vi "Colour.vi"(9 "result":string, 11 "colourRef":refnum<vi>) -> (3 "colourRef 2":refnum<vi>)   [LabVIEW 2020]
panel:
  in  "黄灯":bool
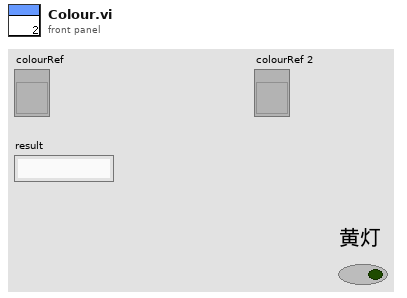
[diagram p1: front panel]
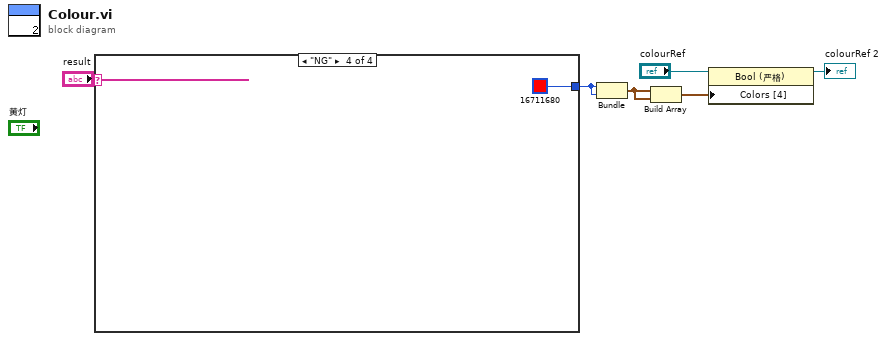
[diagram p0: block diagram]
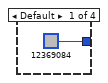
[diagram p2: hidden frame]
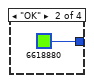
[diagram p3: hidden frame]
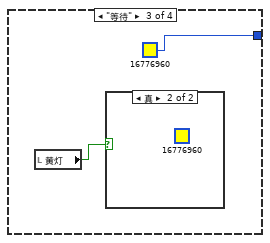
[diagram p4: hidden frame]
diagram:
  n1 = case shown="\"NG\"" "result" {
    tunnel: [u32 12369084 u32 6618880 u32 16776960 u32 16711680] -> w6
    frame Default {
    }
    frame "OK" {
    }
    frame "等待" {
      n2 = local read "黄灯"() -> (w10:bool)
      n3 = case shown="真" w10 {
        frame False {
        }
        frame True {
          (unwired) u32 16776960
        }
      }
    }
    frame "NG" {
    }
  }
  n4 = Bundle(w6, w6) -> (w5:cluster{u32, u32})  [unwired: 1 in]
  n5 = Build Array(w5, w5) -> (w1:cluster{u32, u32}[])
  n6 = property class="Bool (严格)"(reference="colourRef", "Colors [4]"=w1) -> (reference out=→"colourRef 2":refnum<vi>)  [unwired: 1 in, 1 out]
